vi "Pin Name.vi"() -> (2 "Pin Name":string="niDCPower")   [LabVIEW 2021, in "Migrator Reusables.lvlib"]
uses:
  Migrator Reusables.lvlib
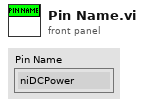
[diagram p1: front panel]
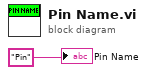
[diagram p0: block diagram]
diagram:
  "Pin Name" <- "Pin" ("Pin Name")
